vi "test_LoadCommandlineArgs_ActiveTarget.vi"() -> (3 "Pass?":bool)   [LabVIEW 2019, in "Tests.SolutionBuilder.lvlib"]
uses:
  Tests.SolutionBuilder.lvlib
  SolutionBuilder/Community/Options.ctl
  SolutionBuilder/SolutionBuilder.lvclass
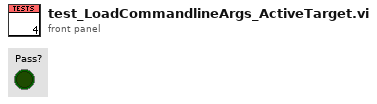
[diagram p1: front panel]
types:
  T1 = typedef "SolutionBuilder.lvlib/SolutionBuilder.lvclass/Options.ctl" = cluster{"Path":path, "Preview?":bool, "Quiet?":bool, "Log file":path, "Success file":path, "Rebuild?":bool, "Keep split projects?":bool}
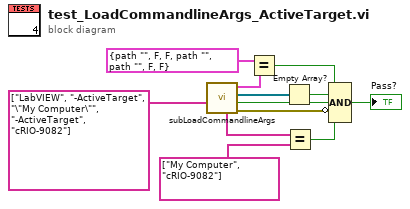
[diagram p0: block diagram]
diagram:
  n1 = call "subLoadCommandlineArgs.vi"("App.Args"=string[] ["LabVIEW", "-ActiveTarget", "\"My Computer\"", "-ActiveTarget", "cRIO-9082"]) -> ("error out"=w10:errorcluster, "From command line?"=w5:bool, "Pre-built libraries"=w8:refnum<class "ProjectItem.lvclass">[], "Options"=w9:T1, "Active targets"=w4:string[])  [unwired: 6 in]
  n2 = Equal?(x=T1 {"Path"=path "", "Preview?"=FALSE, "Quiet?"=FALSE, "Log file"=path "", "Success file"=path "", "Rebuild?"=FALSE, "Keep split projects?"=FALSE} ("Options"), y=w9) -> (x = y?=w6:bool)
  n3 = Empty Array?(array=w8) -> (empty?=w7:bool)
  n4 = Equal?(x=w4, y=string[] ["My Computer", "cRIO-9082"]) -> (x = y?=w2:bool)
  n5 = Compound Arithmetic op=AND(w6, w7, w5, invert w10, w2) -> (→"Pass?":bool)
